vi "labVIEW_program.vi"() -> ()   [LabVIEW 2020]
uses:
  <vilib>/Instr/_visa.llb/VISA Configure Serial Port (Instr).vi
panel:
  out "unsigned byte array":u8[](array[numeric])
  in  "MICRO":dbl(slide) scale=0.0..255.0
  out "LECTURA ADC":i32(graph)
  in  "stop":bool
  in  "PUERTO":refnum<visa-resource-name>
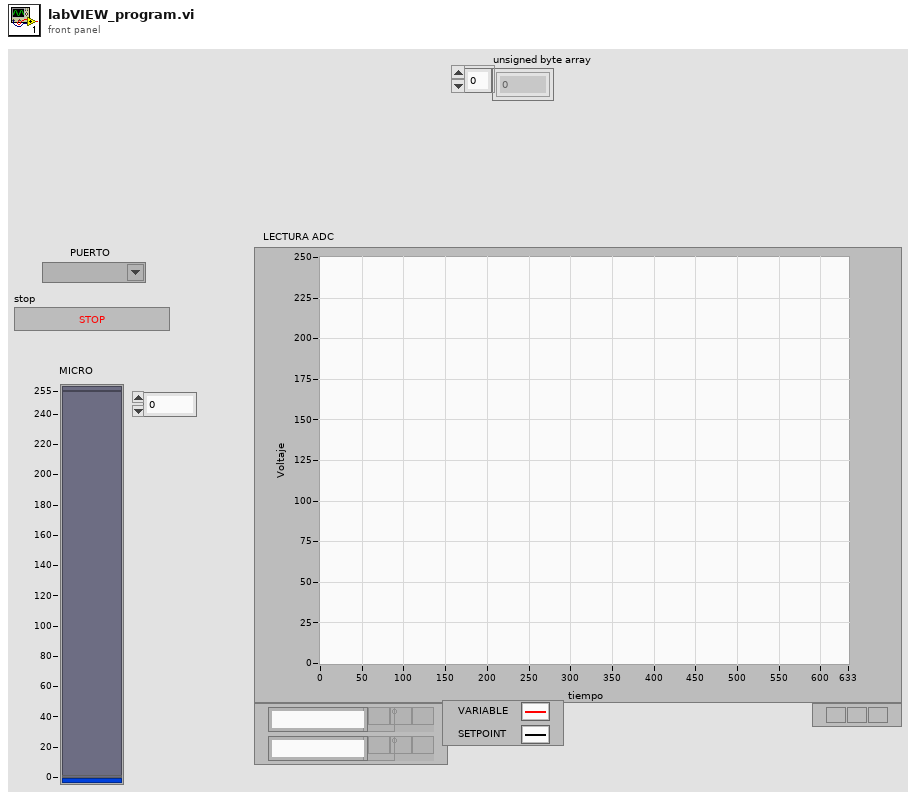
[diagram p1: front panel]
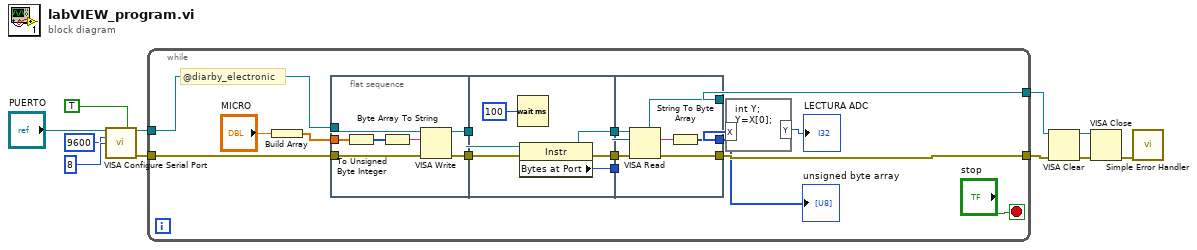
[diagram p0: block diagram]
diagram:
  n1 = call-poly "VISA Configure Serial Port"("VISA resource name"="PUERTO", "Enable Termination\nChar (T)"=TRUE ("Enable Termination\nChar (T)"), "baud rate (9600)"=u32 9600, "data bits (8)"=u16 8) -> ("VISA resource name out"=w4:refnum<visa-resource-name>, "error out"=w3:errorcluster)  [unwired: 10 in]
  n2 = while {
    tunnel: [w22] -> w10
    tunnel: [w21] -> w7
    tunnel: w4 -> [w20]
    tunnel: w3 -> [w19]
    stop <- "stop" stop-if-true
    # "@diarby_electronic"
    n3 = Build Array("MICRO") -> (w18:dbl[])
    n4 = flat-sequence {
      tunnel: [w32] -> w25
      tunnel: [w31] -> w24
      tunnel: w20 -> [w29]
      tunnel: w19 -> [w28]
      tunnel: w18 -> [w27]
      tunnel: w25 -> [w37]
      tunnel: w24 -> [w36]
      tunnel: [w35] -> w14
      tunnel: [w34] -> w13
      tunnel: [w33] -> w12
      tunnel: [w45] -> w22
      tunnel: [w44] -> w21
      tunnel: [w42] -> w17
      tunnel: w14 -> [w41]
      tunnel: w13 -> [w40]
      tunnel: w12 -> [w39]
      frame #0 {
        n5 = To Unsigned Byte Integer(number=w27) -> (unsigned 8bit integer=w26:u8[])
        n6 = Byte Array To String(unsigned byte array=w26) -> (string=w30:string)
        n7 = VISA Write(VISA resource name=w29, write buffer=w30, error in (no error)=w28) -> (VISA resource name out=w32:refnum<visa-resource-name>, error out=w31:errorcluster)  [unwired: 1 out]
      }
      frame #1 {
        n8 = Wait (ms)(milliseconds to wait=u32 100) -> ()  [unwired: 1 out]
        n9 = property class="Instr"(reference=w37, error in=w36) -> (reference out=w35:refnum<visa-resource-name>, error out=w33:errorcluster, "Bytes at Port"=w34:u32)
      }
      frame #2 {
        n10 = VISA Read(VISA resource name=w41, byte count=w40, error in (no error)=w39) -> (VISA resource name out=w44:refnum<visa-resource-name>, read buffer=w43:string, error out=w45:errorcluster)  [unwired: 1 out]
        n11 = String To Byte Array(string=w43) -> (unsigned byte array=w42:u8[])
      }
    }
    n12 = formula code="int Y;\nY=X[0];"("X"=w17) -> ("Y"=→"LECTURA ADC":i32)
    "unsigned byte array" <- w17
  }
  n13 = VISA Clear(VISA resource name=w7, error in (no error)=w10) -> (VISA resource name out=w9:refnum<visa-resource-name>, error out=w8:errorcluster)
  n14 = VISA Close(VISA resource name=w9, error in (no error)=w8) -> (error out=w11:errorcluster)
  n15 = call <vilib>:"Simple Error Handler.vi"("error in (no error)"=w11) -> ()  [unwired: 1 in, 8 out]
